vi "Set Ac Dc.vi"(8 "error in (no error)":errorcluster, 10 "ac":i32, 11 "channel":u32) -> (0 "error out":errorcluster)   [LabVIEW 2021, in "vmmso.lvlib"]
doc: "DLL_API void WINAPI SetAcDc(unsigned int channel, int ac);"
uses:
  vmmso.lvlib
  vmmso.dll
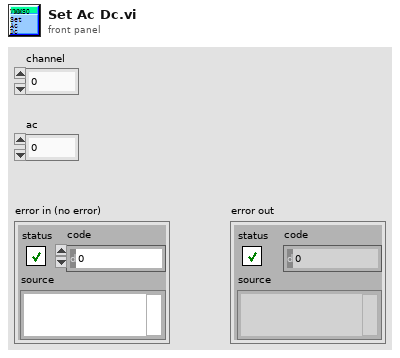
[diagram p1: front panel]
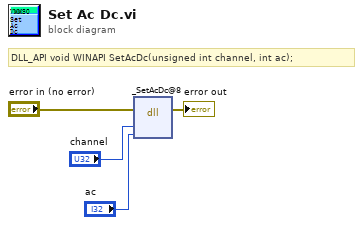
[diagram p0: block diagram]
diagram:
  # "DLL_API void WINAPI SetAcDc(unsigned int channel, int ac);"
  n1 = dll-call lib="O:/MSO/library/demo-Labview/vmmso/vmmso.*" fn="_SetAcDc@8"(error in="error in (no error)", "channel"="channel", "ac"="ac") -> (error out=→"error out":errorcluster)  [unwired: 5 in, 1 out]
